vi "Process Raster Data.vi"(11 "Input Array":cluster{dbl[unit], dbl[]}[](array[cluster])) -> (1 "Avg Counts":dbl[](array[numeric]), 2 "Raw counts":i32[][](array[numeric]), 3 "Wavelengths":dbl[](array[numeric]))   [LabVIEW 2017, in "Synapse CCD.lvclass"]
uses:
  Synapse CCD.lvclass
panel:
  in  "stop":bool
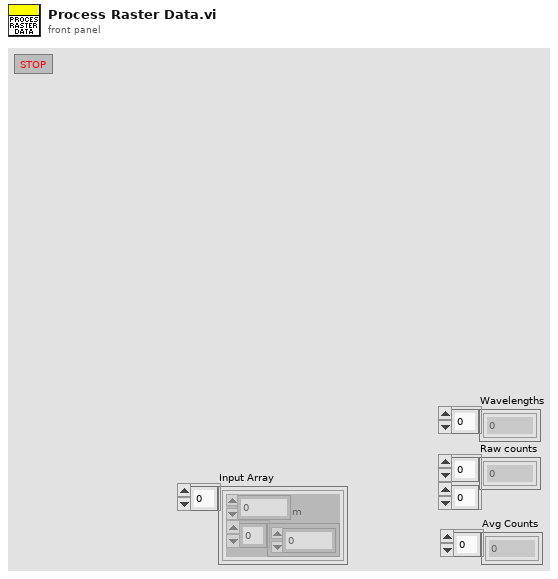
[diagram p1: front panel]
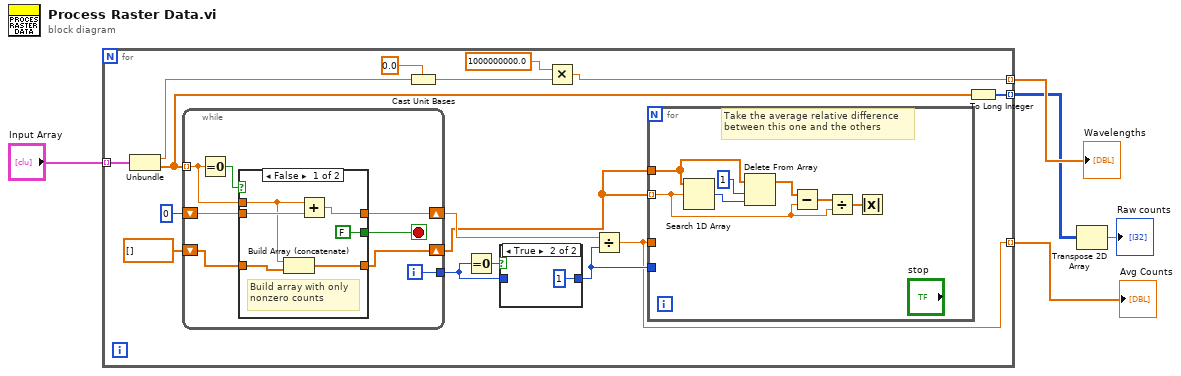
[diagram p0: block diagram]
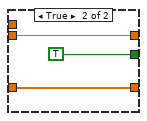
[diagram p3: hidden frame]
diagram:
  n1 = for {
    tunnel: "Input Array" -> [w21] mode=indexing
    tunnel: [w10] -> w3 mode=indexing
    tunnel: [w7] -> w4 mode=indexing
    tunnel: [w15] -> w1 mode=indexing
    n2 = Unbundle(w21) -> (w18:dbl[unit], w13:dbl[])
    n3 = while {
      tunnel: w13 -> [w35] mode=indexing
      shift-right: [w34] -> w19
      shift-left: 0 -> [w36]
      tunnel: [w33] -> w16
      shift-right: [w32] -> w11
      shift-left: dbl[] [] -> [w31]
      i -> [w33]
      stop <- w37 stop-if-true
      n4 = Equal To 0?(x=w35) -> (x = 0?=w38:bool)
      n5 = case shown="False" w38 {
        tunnel: [FALSE TRUE] -> w37
        tunnel: w36 -> [w44 w46]
        tunnel: w35 -> [w41 _]
        tunnel: [w43 w46] -> w34
        tunnel: [w40 w45] -> w32
        tunnel: w31 -> [w39 w45]
        frame False {
          # "Build array with only\nnonzero counts"
          n6 = Build Array (concatenate)(w41, w39) -> (w40:dbl[])
          n7 = Add(x=w41, y=w44) -> (x+y=w43:dbl)
        }
        frame True {
        }
      }
    }
    n8 = Cast Unit Bases(0:w18, 1:0.0 ("unit (none)")) -> (2:w9:dbl)
    n9 = Equal To 0?(x=w16) -> (x = 0?=w17:bool)
    n10 = case shown="True" w17 {
      tunnel: w16 -> [w29 _]
      tunnel: [w29 1] -> w14
      frame False {
      }
      frame True {
      }
    }
    n11 = Multiply(x=1000000000.0, y=w9) -> (x*y=w7:dbl)
    n12 = Divide(x=w19, y=w14) -> (x/y=w10:dbl)
    n13 = for {
      tunnel: w10 -> [_]
      tunnel: w14 -> [_]
      tunnel: w11 -> [w23] mode=indexing
      tunnel: w11 -> [w28]
      # "Take the average relative difference \nbetween this one and the others"
      n14 = Search 1D Array(1D array=w28, element=w23) -> (index of element=w26:i32)  [unwired: 1 in]
      n15 = Delete From Array(array=w28, length=1, index=w26) -> (array with subset deleted=w25:dbl[])  [unwired: 1 out]
      n16 = Subtract(x=w25, y=w23) -> (x-y=w24:dbl[])
      n17 = Divide(x=w24, y=w23) -> (x/y=w22:dbl[])
      n18 = Absolute Value(x=w22) -> ()  [unwired: 1 out]
    }
    n19 = To Long Integer(number=w13) -> (32bit integer=w15:i32[])
  }
  "Wavelengths" <- w4
  "Avg Counts" <- w3
  n20 = Transpose 2D Array(2D array=w1) -> (transposed array=→"Raw counts":i32[][])
